vi "InitBase.vi"(5 "FPGA refs":refnum<class "FpgaRefBase.lvclass">[](array[class]), 6 "RemoteConnection":refnum<class "RemoteConnection.lvclass">, 7 "Chart length":i32, 8 "Trigger":T1, 9 "data mode":T2, 10 "Samples Per Trigger":i32=5000000, 11 "ScopeBase in":refnum<class "ScopeBase.lvclass">) -> (0 "error out":errorcluster, 3 "ScopeBase out":refnum<class "ScopeBase.lvclass">)   [LabVIEW 2013, in "ScopeBase.lvclass"]
uses:
  ScopeBase.lvclass
  FPGA/DataMode.ctl
  Scope5782/Scope/controls/5782_trigger_type.ctl
  Communication/Driver/RemoteConnection/RemoteConnection.lvclass
  FpgaRef/FpgaRefBase/FpgaRefBase.lvclass
  controls/ScopeMode.ctl
  FPGA/fpga_settings.ctl
  ScopeBase.lvclass/ScopeBase.ctl
  <vilib>/rvi/FXPMathLib/FxpInterpret/XNode/nifxpmath_Interpret.xnode
  Utilities/Ticker/Ticker.lvclass
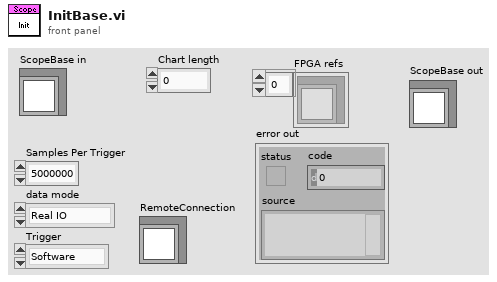
[diagram p1: front panel]
types:
  T1 = typedef "5782_trigger_type.ctl" = enum16{"Software", "Trigger input"}
  T2 = typedef "DataMode.ctl" = enum16{"Real IO", "Simulated"}
  T3 = typedef "fpga_settings.ctl" = enum16{"Feedback Enable", "New FIR coeffs", "FIR shift", "Enable filter", "Set Downsample", "Downsample", "CIC Gain", "Record length", "Trigger samples", "Quiet time", "a_am", "b_am", "Use fixed delay", "fixed sin_fi", "fixed cos_fi", "Ki*Tau", "Kp", "Kd_Tau", "Fi_start", "Fi_delta", "DC_offs 0", "DC_offs 1", "DC_offs 2", "DC_offs 3", "Ki*Tau am", "Kp am", "Kd_Tau am", "Feedback AM", "Trigger delay", "Feedback delay", "Setpoint enable", "Beam enable", "Samples to acquire", "Cavity Enable"}
  T4 = typedef "ScopeMode.ctl" = enum16{"Stopped", "Single", "Running", "Continuous"}
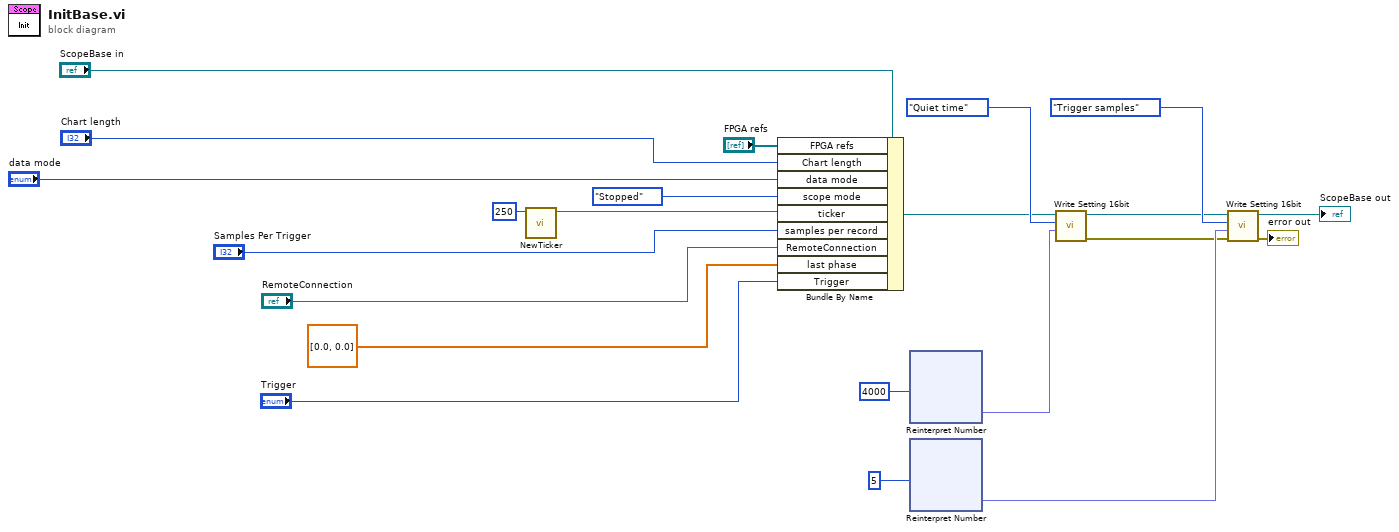
[diagram p0: block diagram]
diagram:
  n1 = call "NewTicker.vi"("Period"=u32 250) -> ("Ticker"=w20:refnum<class "Ticker.lvclass">)  [unwired: 10 in]
  n2 = Bundle By Name(cluster="ScopeBase in", "FPGA refs"="FPGA refs", "Chart length"="Chart length", "data mode"="data mode", "scope mode"=ScopeMode."Stopped", "ticker"=w20, "samples per record"="Samples Per Trigger", "RemoteConnection"="RemoteConnection", "last phase"=dbl[] [0.0, 0.0], "Trigger"="Trigger") -> (w7:refnum<class "ScopeBase.lvclass">)
  n3 = xnode "Reinterpret Number"("x"=u16 4000 ("Samples to aqcuire")) -> ("y"=w4:fxp<+,16,16>)
  n4 = xnode "Reinterpret Number"("x"=u16 5 ("trigger samples")) -> ("y"=w3:fxp<+,16,16>)
  n5 = call "Write Setting 16bit.vi"("value"=w4, "FPGA Setting"=fpga_settings."Quiet time", "ScopeBase in"=w7) -> ("error out"=w2:errorcluster, "ScopeBase out"=w10:refnum<class "ScopeBase.lvclass">)  [unwired: 7 in]
  n6 = call "Write Setting 16bit.vi"("error in (no error)"=w2, "value"=w3, "FPGA Setting"=fpga_settings."Trigger samples", "ScopeBase in"=w10) -> ("error out"=→"error out":errorcluster, "ScopeBase out"=→"ScopeBase out":refnum<class "ScopeBase.lvclass">)  [unwired: 6 in]
